vi "Enable Data Stream.vi"(8 "error in (no error)":errorcluster, 9 "Message Interval (hz)":u16=10, 10 "req_stream_id":T1(ring)=enum."RAW_SENSORS", 11 "Aircraft Index":u8) -> (0 "error out":errorcluster)   [LabVIEW 2014]
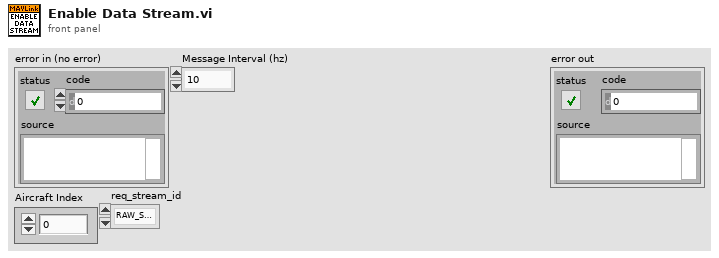
[diagram p1: front panel]
types:
  T1 = enum16{"ALL", "RAW_SENSORS", "EXTENDED_STATUS", "RC_CHANNELS", "RAW_CONTROLLER", "POSITION", "EXTRA1", "EXTRA2", "EXTRA3"}
  T2 = cluster{"req_message_rate":u16, "target_system":u8, "target_component":u8, "req_stream_id":enum16{"ALL", "RAW_SENSORS", "EXTENDED_STATUS", "RC_CHANNELS", "RAW_CONTROLLER", "POSITION", "EXTRA1", "EXTRA2", "EXTRA3"}, "start_stop":bool}
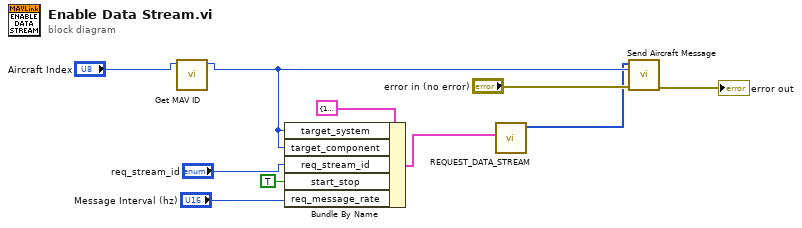
[diagram p0: block diagram]
diagram:
  n1 = call "Get MAV ID.vi"("Aircraft Index"="Aircraft Index") -> ("Aircraft ID"=w6:u8)  [unwired: 9 in, 1 out]
  n2 = Bundle By Name(cluster=T2 {"req_message_rate"=10, "target_system"=0, "target_component"=0, "req_stream_id"=enum."ALL", "start_stop"=FALSE} ("Payload"), "target_system"=w6, "target_component"=w6, "req_stream_id"="req_stream_id", "start_stop"=TRUE, "req_message_rate"="Message Interval (hz)") -> (w5:T2)
  n3 = call "REQUEST_DATA_STREAM.vi"("Payload"=w5) -> ("MAVLink MSG"=w4:u8[])  [unwired: 10 in]
  n4 = call "Send Aircraft Message.vi"("error in (no error)"="error in (no error)", "Aircraft ID"=w6, "MAVLink Message"=w4) -> ("error out"=→"error out":errorcluster)  [unwired: 8 in]
